vi "H5Fcreate.vi"(2 "filename":path, 7 "flags":T1[](array[typedef]), 9 "error in (no error)":errorcluster) -> (0 "file_id":i32, 6 "error out":errorcluster)   [LabVIEW 2009]
uses:
  H5F_ACC.ctl
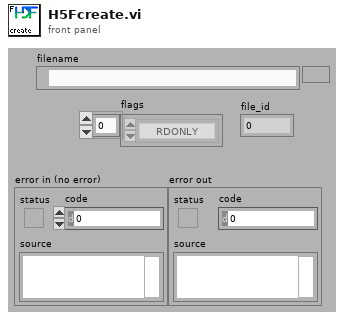
[diagram p1: front panel]
types:
  T1 = typedef "H5F_ACC.ctl" = enum16{"RDONLY", "RDWR", "TRUNC", "EXCL", "DEBUG", "CREAT"}
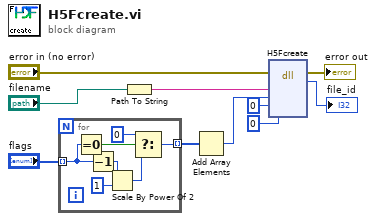
[diagram p0: block diagram]
diagram:
  n1 = for {
    tunnel: "flags" -> [w16] mode=indexing
    tunnel: [w12] -> w6 mode=indexing
    n2 = Equal To 0?(x=w16) -> (x = 0?=w15:bool)
    n3 = Decrement(x=w16) -> (x-1=w11:T1)
    n4 = Scale By Power Of 2(n=w11, x=u32 1) -> (x*2^n=w13:u32)
    n5 = Select(t=u32 0, s=w15, f=w13) -> (s? t:f=w12:u32)
  }
  n6 = Path To String(path="filename") -> (string=w2:string)
  n7 = Add Array Elements(numeric array=w6) -> (sum=w5:u32)
  n8 = dll-call lib="hdf5dll" fn="H5Fcreate"(error in="error in (no error)", "filename"=w2, "flags"=w5, "create_plist"=0, "access_plist"=0) -> (error out=→"error out":errorcluster, "return type"=→"file_id":i32)  [unwired: 6 in, 1 out]
